vi "terminate.vi"(8 "error in (no error)":errorcluster, 11 "DAQmxAnalogOut in":refnum<class "AnalogOutDL101207DAQmx.lvclass">) -> (0 "error out":errorcluster, 3 "DAQmxAnalogOut out":refnum<class "AnalogOutDL101207DAQmx.lvclass">)   [LabVIEW 2010, in "AnalogOutDL101207DAQmx.lvclass"]
doc: "The dynamic dispatch version of this VI terminates the plug-in object by releasing all of its resources."
uses:
  AnalogOutDL101207DAQmx.lvclass
  AnalogOutDL101207DAQmx.lvclass/AnalogOutDL101207DAQmx.ctl
  GenericAnalogOut/GenericAnalogOut/GenericAnalogOut.lvclass
  common/classes/ErrorController/ErrorController/class_data.vi
  common/classes/ErrorController/ErrorController/ErrorController.lvclass
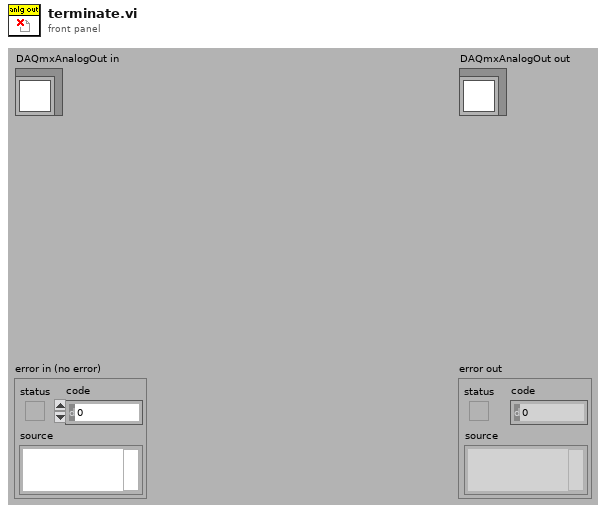
[diagram p1: front panel]
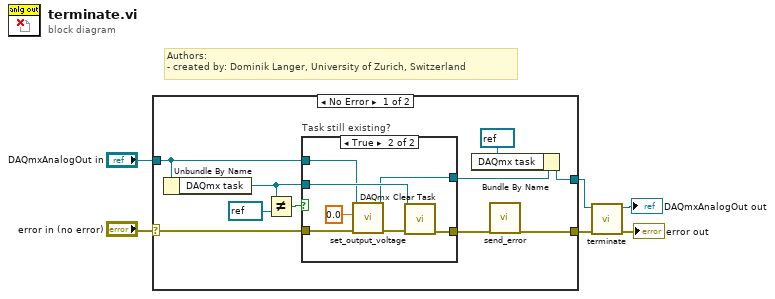
[diagram p0: block diagram]
diagram:
  # "Authors: \n- created by: Dominik Langer, University of Zurich, Switzerland"
  n1 = case shown="No Error" "error in (no error)" {
    selector: "error in (no error)" -> [w12 w27]
    tunnel: "DAQmxAnalogOut in" -> [w11 w26]
    tunnel: [w8 w27] -> w2
    tunnel: [w9 w26] -> w1
    frame No Error {
      n2 = Unbundle By Name(w11) -> ("DAQmx task"=w15:refnum<k21>)
      n3 = Not Equal?(x=w15, y=refnum<k21> refnum ("shutter task")) -> (x != y?=w14:bool)
      n4 = case "Task still existing?" shown="True" w14 {
        tunnel: w12 -> [w17 w23]
        tunnel: w11 -> [w18 w21]
        tunnel: [w18 w20] -> w10
        tunnel: w15 -> [_ w25]
        tunnel: [w17 w24] -> w7
        frame False {
        }
        frame True {
          n5 = call-dynamic "set_output_voltage.vi"("error in (no error)"=w23, "output value"=dbl[unit] 0.0, "DAQmxAnalogOut in"=w21) -> ("error out"=w22:errorcluster, "DAQmxAnalogOut out"=w20:refnum<class "AnalogOutDL101207DAQmx.lvclass">)  [unwired: 7 in]
          n6 = call <vilib>:"DAQmx Clear Task.vi"("task in"=w25, "error in"=w22) -> ("error out"=w24:errorcluster)  [unwired: 13 out]
        }
      }
      n7 = Bundle By Name(cluster=w10, "DAQmx task"=refnum<k21> refnum ("shutter task")) -> (w9:refnum<class "AnalogOutDL101207DAQmx.lvclass">)
      n8 = call "send_error.vi"("error in (no error)"=w7) -> ("error out"=w8:errorcluster)  [unwired: 10 in]
    }
    frame Error {
    }
  }
  n9 = call-parent "terminate.vi"("error in (no error)"=w2, "GenericPlugin in"=w1) -> ("error out"=→"error out":errorcluster, "GenericPlugin out"=→"DAQmxAnalogOut out":refnum<class "AnalogOutDL101207DAQmx.lvclass">)  [unwired: 8 out]
